vi "温度自动滚条.vi"(0 "温度输入1":dbl, 1 "移位输入1":string[][](array[string]), 5 "温度输入 2":dbl, 7 "温度输入 3":dbl, 9 "历史最高":dbl, 11 "历史最低":dbl, 12 "移位输入2":dbl, 13 "行数":dbl, 14 "计数":dbl) -> (4 "移位输出1":string[][](array[string]), 6 "移位输出2":dbl, 8 "表格输出":string[][](table), 10 "温度簇":T1, 15 "簇输出":T2 caption="输出簇")   [LabVIEW 2012]
uses:
  <vilib>/Utility/miscctls.llb/LVRowAndColumnUnsignedTypeDef.ctl
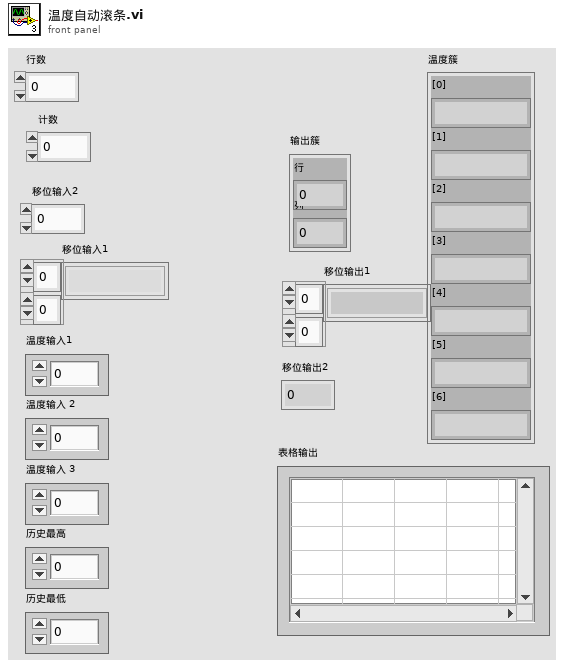
[diagram p1: front panel]
types:
  T1 = cluster{"[0]":string, "[1]":string, "[2]":string, "[3]":string, "[4]":string, "[5]":string, "[6]":string}
  T2 = typedef "LVRowAndColumnUnsignedTypeDef.ctl" = cluster{"Row":u32, "Column":u32}
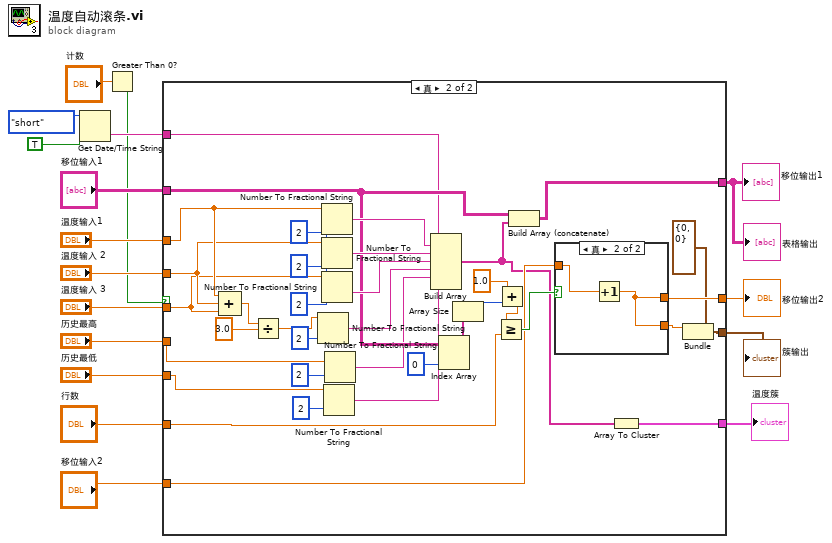
[diagram p0: block diagram]
diagram:
  n1 = Get Date/Time String(date format (0)=enum16{"short", "long", "abbreviated"}."short" ("日期格式(0)"), want seconds? (F)=TRUE ("需要秒？(F)")) -> (time string=w6:string)  [unwired: 1 in, 1 out]
  n2 = Greater Than 0?(x="计数") -> (x > 0?=w4:bool)
  n3 = case shown="真" w4 {
    tunnel: [_ w49] -> w17
    tunnel: "历史最高" -> [_ w43]
    tunnel: "温度输入 2" -> [_ w28]
    tunnel: "温度输入 3" -> [_ w27]
    tunnel: "移位输入2" -> [_ w42]
    tunnel: "移位输入1" -> [_ w41]
    tunnel: [_ w39] -> w11
    tunnel: [_ w38] -> w10
    tunnel: "行数" -> [_ w37]
    tunnel: "温度输入1" -> [_ w29]
    tunnel: w6 -> [_ w36]
    tunnel: "历史最低" -> [_ w32]
    tunnel: [_ w18] -> w2
    frame False {
    }
    frame True {
      n4 = Compound Arithmetic op=ADD(w29, w28, w27) -> (w26:dbl)
      n5 = Divide(x=w26, y=3.0) -> (x/y=w24:dbl)
      n6 = Number To Fractional String(number=w24, precision (6)=i16 2 ("精度(6)")) -> (F-format string=w22:string)  [unwired: 2 in]
      n7 = Number To Fractional String(number=w29, precision (6)=i16 2 ("精度(6)")) -> (F-format string=w47:string)  [unwired: 2 in]
      n8 = Number To Fractional String(number=w28, precision (6)=i16 2 ("精度(6)")) -> (F-format string=w45:string)  [unwired: 2 in]
      n9 = Number To Fractional String(number=w27, precision (6)=i16 2 ("精度(6)")) -> (F-format string=w44:string)  [unwired: 2 in]
      n10 = Number To Fractional String(number=w32, precision (6)=i16 2 ("精度(6)")) -> (F-format string=w20:string)  [unwired: 2 in]
      n11 = Number To Fractional String(number=w43, precision (6)=i16 2 ("精度(6)")) -> (F-format string=w21:string)  [unwired: 2 in]
      n12 = Build Array(w36, w47, w45, w44, w22, w21, w20) -> (w19:string[])
      n13 = Index Array(array=w41, index (col)=0 ("索引")) -> (element=w54:string[])  [unwired: 1 in]
      n14 = Array Size(array=w54) -> (size(s)=w52:i32)
      n15 = Add(x=1.0, y=w52) -> (x+y=w51:dbl)
      n16 = Greater Or Equal?(x=w51, y=w37) -> (x >= y?=w50:bool)
      n17 = Build Array (concatenate)(w41, w19) -> (w39:string[][])
      n18 = case shown="真" w50 {
        tunnel: w42 -> [w55 w56]
        tunnel: [w55 w57] -> w49
        tunnel: [_ w57] -> w48
        frame False {
        }
        frame True {
          n19 = Increment(x=w56) -> (x+1=w57:dbl)
        }
      }
      n20 = Array To Cluster(array=w19) -> (cluster=w18:T1)
      n21 = Bundle(cluster=T2 {"Row"=0, "Column"=0} ("索引值"), "Row"=w48) -> (w38:T2)  [unwired: 1 in]
    }
  }
  "移位输出2" <- w17
  "移位输出1" <- w11
  "表格输出" <- w11
  "簇输出" <- w10
  "温度簇" <- w2
